vi "Read Device 1.vi"(8 "error in (no error)":errorcluster, 11 "AlicatPressureController in":refnum<class "AlicatPressureController.lvclass">) -> (0 "error out":errorcluster, 3 "AlicatPressureController out":refnum<class "AlicatPressureController.lvclass">)   [LabVIEW 2020, in "AlicatPressureController.lvclass"]
uses:
  AlicatPressureController.lvclass
  AlicatPressureController.lvclass/AlicatPressureController.ctl
  OnOffTypeDef.ctl
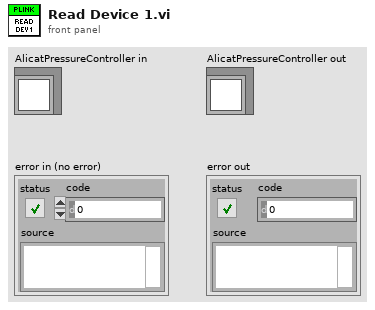
[diagram p1: front panel]
types:
  T1 = typedef "OnOffTypeDef.ctl" = enum16{"off", "on"}
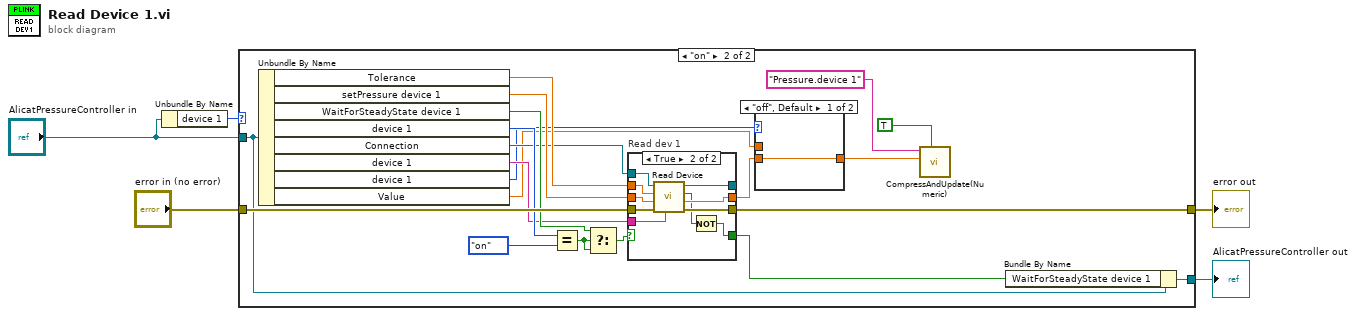
[diagram p0: block diagram]
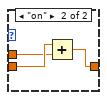
[diagram p3: hidden frame]
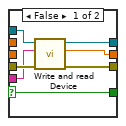
[diagram p4: hidden frame]
diagram:
  n1 = Unbundle By Name("AlicatPressureController in") -> ("device 1"=w2:T1)
  n2 = case shown="\"on\"" w2 {
    tunnel: "error in (no error)" -> [w7 w27]
    tunnel: [w6 w8] -> w5
    tunnel: [w7 w26] -> w1
    tunnel: "AlicatPressureController in" -> [w6 w9]
    frame "off", Default {
    }
    frame "on" {
      n3 = Unbundle By Name(w9) -> ("Tolerance"=w22:dbl, "setPressure device 1"=w21:dbl, "WaitForSteadyState device 1"=w20:bool, "device 1"=w19:T1, "Connection"=w18:refnum<visa-resource-name>, "device 1"=w17:string, "device 1"=w15:T1, "Value"=w11:dbl)
      n4 = Equal?(x=w19, y=OnOffTypeDef."on") -> (x = y?=w24:bool)
      n5 = Select(t=w20, s=w24, f=w24) -> (s? t:f=w23:bool)
      n6 = case "Read dev 1" shown="True" w23 {
        selector: w23 -> [w32 _]
        tunnel: w27 -> [w38 w48]
        tunnel: [w34 w47] -> w26
        tunnel: [w35 w46] -> _
        tunnel: [w33 w45] -> w16
        tunnel: w18 -> [w36 w44]
        tunnel: w17 -> [w37 w40]
        tunnel: w21 -> [_ w42]
        tunnel: w22 -> [_ w43]
        tunnel: [w32 w39] -> w10
        frame False {
          n7 = call "Write and read Device.vi"("error in (no error)"=w38, "device 1"=w37, "VISA Refnum in"=w36) -> ("error out"=w34:errorcluster, "pressure reading"=w33:dbl, "VISA Refnum out"=w35:refnum<visa-resource-name>)  [unwired: 5 in, 1 out]
        }
        frame True {
          n8 = call "Read Device.vi"("device address"=w40, "error in (no error)"=w48, "setPressure"=w42, "Tolerance"=w43, "VISA Refnum in"=w44) -> ("error out"=w47:errorcluster, ">Reading in native controller units>"=w45:dbl, "Boolean"=w41:bool, "VISA Refnum out"=w46:refnum<visa-resource-name>)  [unwired: 3 in]
          n9 = Not(x=w41) -> (.not. x?=w39:bool)
        }
      }
      n10 = case shown="\"off\", Default" w15 {
        tunnel: w16 -> [w28 w31]
        tunnel: [w28 w30] -> w12
        tunnel: w11 -> [_ w29]
        frame "off", Default {
        }
        frame "on" {
          n11 = Add(x=w31, y=w29) -> (x+y=w30:dbl)
        }
      }
      n12 = call "CompressAndUpdate(Numeric).vi"("force CVT update (false)"=TRUE, "Numeric"=w12, "command or variable name"="Pressure.device 1") -> ()  [unwired: 8 in, 1 out]
      n13 = Bundle By Name(cluster=w9, "WaitForSteadyState device 1"=w10) -> (w8:refnum<class "AlicatPressureController.lvclass">)
    }
  }
  "AlicatPressureController out" <- w5
  "error out" <- w1
